vi "Scale Channel (Array).vi"(9 "Data":dbl[](array[numeric]), 10 "Scaling Params":dbl[](array[numeric]), 11 "Scaling Type":T1) -> (1 "Scaled Data":dbl[](array[numeric]))   [LabVIEW 2020, in "VolatusData.lvlib" / "Scaling.lvclass"]
uses:
  Scaling.lvclass
  VolatusConfig/Scale Type.ctl
  Scaling.lvclass/Scaling.ctl
  VolatusConfig/VolatusConfig.lvlib
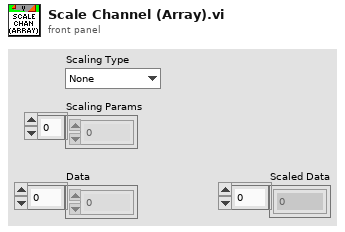
[diagram p1: front panel]
types:
  T1 = typedef "VolatusConfig.lvlib/Scale Type.ctl" = enum16{"None", "Sensor", "Polynomial", "Threshold", "Invert Bool"}
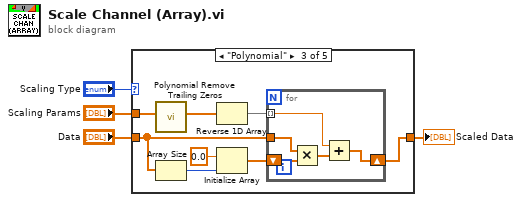
[diagram p0: block diagram]
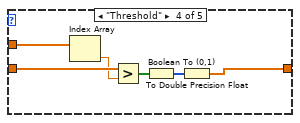
[diagram p4: hidden frame]
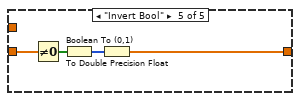
[diagram p5: hidden frame]
diagram:
  n1 = case shown="\"Polynomial\"" "Scaling Type" {
    tunnel: "Scaling Params" -> [_ _ w13 w25 _]
    tunnel: "Data" -> [w5 w6 w9 w24 w29]
    tunnel: [w5 w6 w7 w20 w26] -> w1
    frame "None" {
    }
    frame "Sensor" {
      # "#ERROR?\nSensor should be converted to another type. At least keep raw value passed through to be displayed and logged."
    }
    frame "Polynomial" {
      n2 = call "Polynomial Remove Trailing Zeros.vi"("Coefficients"=w13) -> ("Used Coefficients"=w14:dbl[])  [unwired: 10 in]
      n3 = Array Size(array=w9) -> (size(s)=w12:i32)
      n4 = Reverse 1D Array(array=w14) -> (reversed array=w8:dbl[])
      n5 = Initialize Array(0.0 ("element"), w12) -> (w10:dbl[])
      n6 = for {
        shift-right: [w15] -> w7
        shift-left: w10 -> [w19]
        tunnel: w9 -> [w18]
        tunnel: w8 -> [w16] mode=indexing
        n7 = Multiply(x=w18, y=w19) -> (x*y=w17:dbl[])
        n8 = Add(x=w16, y=w17) -> (x+y=w15:dbl[])
      }
    }
    frame "Threshold" {
      n9 = Index Array(array=w25) -> (element=w23:dbl)  [unwired: 1 in]
      n10 = Greater?(x=w24, y=w23) -> (0:w22:bool[])
      n11 = Boolean To (0,1)(Boolean=w22) -> (0, 1=w21:i16[])
      n12 = To Double Precision Float(number=w21) -> (double precision float=w20:dbl[])
    }
    frame "Invert Bool" {
      n13 = Not Equal To 0?(x=w29) -> (x != 0?=w28:bool[])
      n14 = Boolean To (0,1)(Boolean=w28) -> (0, 1=w27:i16[])
      n15 = To Double Precision Float(number=w27) -> (double precision float=w26:dbl[])
    }
  }
  "Scaled Data" <- w1
